vi "Test MQTT-6.0.0-4.vi"(8 "error in (no error)":errorcluster, 11 "Connection Config":refnum<class "Connection.lvclass">) -> (0 "error out":errorcluster, 3 "Connection Config dup":refnum<class "Connection.lvclass">)   [LabVIEW 2013]
uses:
  <vilib>/LabVIEW Open Source Project/MQTT Connection/MQTT_Connection/Connection/Connection.lvclass
  <vilib>/LabVIEW Open Source Project/MQTT Websockets Connection/MQTT_Websockets/Connection/WebsocketsConnection.lvclass
  <vilib>/addons/_JKI Toolkits/Caraya/classes/Test/Test.lvclass
  <vilib>/addons/_JKI Toolkits/Caraya/classes/Assert/Assert.lvclass
panel:
  out "Return Headers":variant
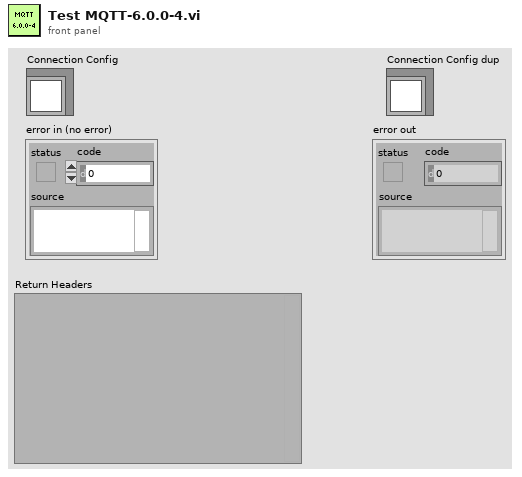
[diagram p1: front panel]
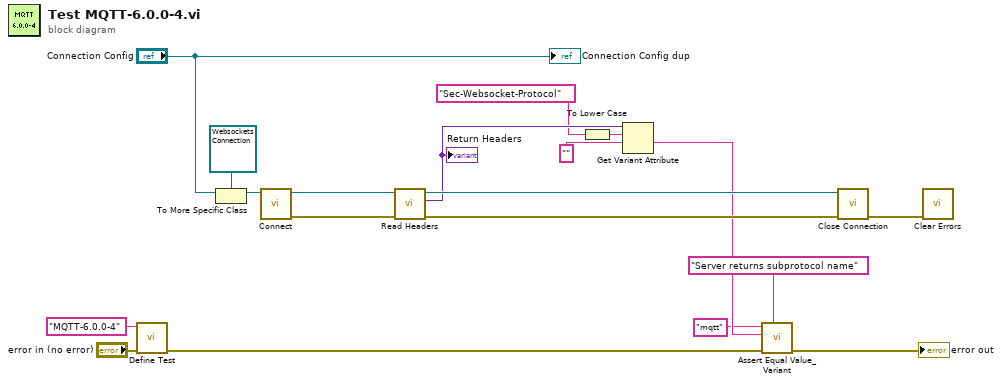
[diagram p0: block diagram]
diagram:
  n1 = call <vilib>:"Define Test.vi"("error in (no error)"="error in (no error)", "Label (VI Title)"="MQTT-6.0.0-4") -> ("error out"=w16:errorcluster)  [unwired: 9 in]
  n2 = To More Specific Class(target class=refnum<class "WebsocketsConnection.lvclass"> refnum ("WebsocketsConnection in"), reference="Connection Config") -> (specific class reference=w13:refnum<class "WebsocketsConnection.lvclass">)  [unwired: 1 in, 1 out]
  n3 = call <vilib>:"Connect.vi"("Connection in"=w13) -> ("error out"=w9:errorcluster, "Connection out"=w10:refnum<class "WebsocketsConnection.lvclass">)  [unwired: 9 in]
  n4 = call <vilib>:"Read Headers.vi"("error in (no error)"=w9, "WebsocketsConnection in"=w10) -> ("error out"=w7:errorcluster, "Return Headers"=w6:variant, "WebsocketsConnection out"=w8:refnum<class "WebsocketsConnection.lvclass">)  [unwired: 7 in]
  "Return Headers" <- w6
  n5 = To Lower Case(string="Sec-Websocket-Protocol" ("name")) -> (all lower case string=w4:string)
  n6 = Get Variant Attribute(Variant=w6, name=w4, default value (empty Variant)="") -> (value=w2:string)  [unwired: 1 in, 3 out]
  n7 = call <vilib>:"Assert Equal Value_Variant.vi"("Label"="Server returns subprotocol name", "error in (no error)"=w16, "Y"=w2, "X"="mqtt") -> ("error out"=→"error out":errorcluster)  [unwired: 7 in]
  n8 = call <vilib>:"Close Connection.vi"("error in (no error)"=w7, "Connection in"=w8) -> ("error out"=w11:errorcluster)  [unwired: 8 in, 1 out]
  n9 = call <vilib>:"Clear Errors.vi"("error in (no error)"=w11) -> ()  [unwired: 6 in, 1 out]
  "Connection Config dup" <- "Connection Config"
